vi "Get egg5302 Formated Parameters.VI"(8 "error in (no error)":errorcluster, 10 "Input String":string, 11 "VISA Resource Name":refnum<visa-resource-name>) -> (0 "error out":errorcluster, 1 "Time Constant":dbl format="%.2e", 2 "Sensitivity":dbl format="%.4e", 3 "Frequency":dbl format="%.2e", 4 "Phase":dbl format="%.2f", 5 "Oscillator voltage":dbl format="%.2e", 6 "Parameters":string, 7 "Data titles":string[](array[string])=["EGG5302_Vx (V)", "EGG5302_Vy (V)"], 9 "VISA Resource Name Out":refnum<visa-resource-name>)   [LabVIEW 2015]
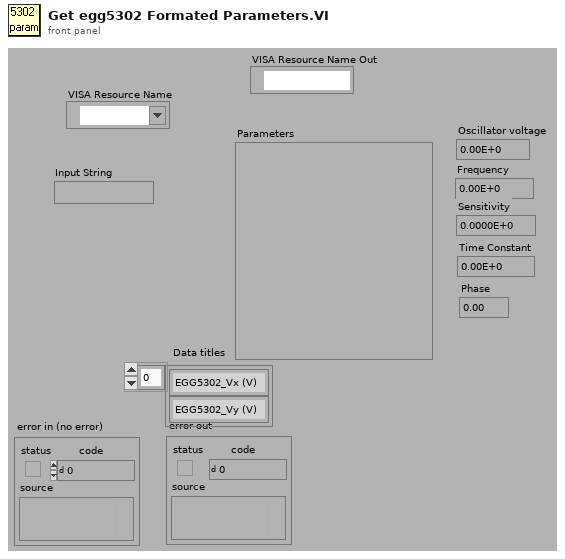
[diagram p1: front panel]
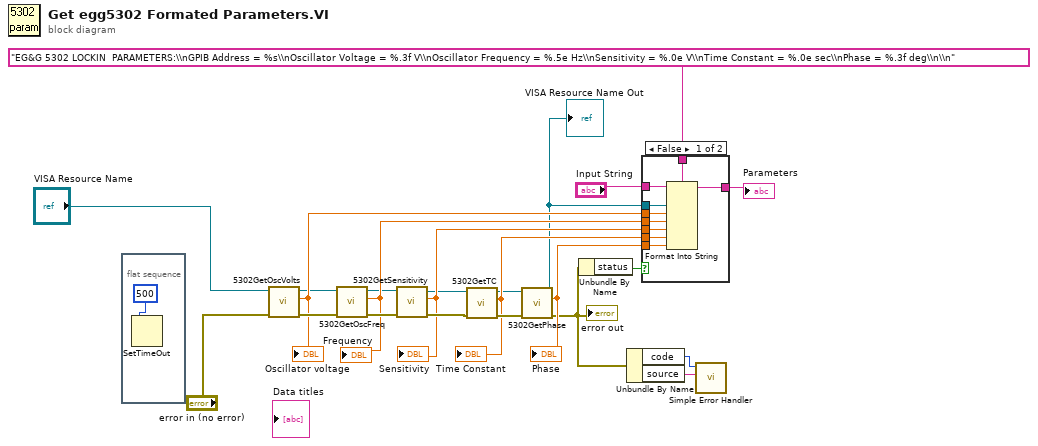
[diagram p0: block diagram]
diagram:
  n1 = flat-sequence {
    frame #0 {
      n2 = SetTimeOut(1:500 ("new timeout (10000)")) -> ()  [unwired: 1 out]
    }
  }
  n3 = call "5302GetOscVolts.vi"("error in (no error)"="error in (no error)", "VISA Resource Name"="VISA Resource Name") -> ("error out"=w23:errorcluster, "Osc Volts"=w15:dbl, "VISA Resource Name Out"=w5:refnum<visa-resource-name>)  [unwired: 1 in, 6 out]
  "Oscillator voltage" <- w15
  n4 = call "5302GetOscFreq.vi"("error in (no error)"=w23, "VISA Resource Name"=w5) -> ("error out"=w22:errorcluster, "Osc Freq"=w16:dbl, "VISA Resource Name Out"=w4:refnum<visa-resource-name>)  [unwired: 1 in, 6 out]
  "Frequency" <- w16
  n5 = call "5302GetSensitivity.vi"("error in (no error)"=w22, "VISA Resource Name"=w4) -> ("error out"=w21:errorcluster, "Sevsitivity"=w17:dbl, "VISA Resource Name Out"=w3:refnum<visa-resource-name>)  [unwired: 1 in, 6 out]
  "Sensitivity" <- w17
  n6 = call "5302GetTC.vi"("error in (no error)"=w21, "VISA Resource Name"=w3) -> ("error out"=w20:errorcluster, "Time Constant"=w18:dbl, "VISA Resource Name Out"=w2:refnum<visa-resource-name>)  [unwired: 1 in, 6 out]
  "Time Constant" <- w18
  n7 = call "5302GetPhase.vi"("error in (no error)"=w20, "VISA Resource Name"=w2) -> ("error out"=w10:errorcluster, "Phase"=w19:dbl, "VISA Resource Name Out"=w1:refnum<visa-resource-name>)  [unwired: 1 in, 6 out]
  "error out" <- w10
  "Phase" <- w19
  "VISA Resource Name Out" <- w1
  n8 = Unbundle By Name(w10) -> ("status"=w13:bool)
  n9 = Unbundle By Name(w10) -> ("code"=w8:i32, "source"=w9:string)
  n10 = case shown="False" w13 {
    tunnel: w19 -> [w33 _]
    tunnel: w18 -> [w32 _]
    tunnel: w17 -> [w31 _]
    tunnel: w16 -> [w30 _]
    tunnel: w15 -> [w29 _]
    tunnel: w1 -> [w28 _]
    tunnel: "EG&G 5302 LOCKIN  PARAMETERS:\\nGPIB Address = %s\\nOscillator Voltage = %.3f V\\nOscillator Frequency = %.5e Hz\\nSensitivity = %.0e V\\nTime Constant = %.0e sec\\nPhase = %.3f deg\\n\\n" -> [w27 _]
    tunnel: "Input String" -> [w26 w34]
    tunnel: [w25 w34] -> w11
    frame False {
      n11 = Format Into String(format string=w27, initial string=w26, w28, w29, w30, w31, w32, w33) -> (resulting string=w25:string)  [unwired: 1 in, 1 out]
    }
    frame True {
    }
  }
  "Parameters" <- w11
  n12 = call <vilib>:"Simple Error Handler.vi"("error code (no error:0)"=w8, "error source (\" \")"=w9) -> ()  [unwired: 2 in, 6 out]
